vi "Финал (5).vi"(0 "Dec":T5, 1 "Cread":bool, 2 "adr A":cluster{"A1":bool, "A0":bool}, 3 "adr B":cluster{"B1":bool, "B0":bool}, 4 "SelInp":bool, 5 "C Func":T1, 6 "SelOp":bool, 7 "Reset Out":bool, 8 "WR":bool, 9 "Reset":bool, 10 "C":bool, 11 "Exec":bool, 12 "Reset Memory":bool, 13 "ClearAcc":bool, 19 "Read":bool) -> (14 "L":T3, 15 "Flags":T4, 16 "Digs":T2)   [LabVIEW 2017]
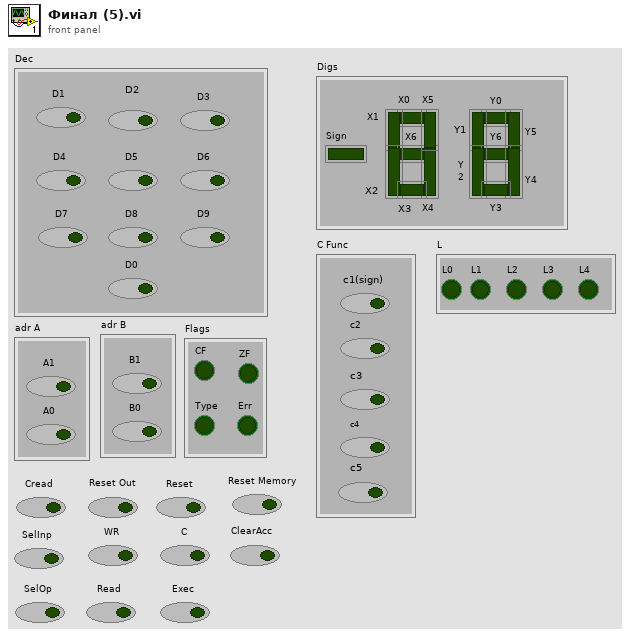
[diagram p1: front panel]
types:
  T1 = cluster{"c1(sign)":bool, "c2":bool, "c3":bool, "c4":bool, "c5":bool}
  T2 = cluster{"Y0":bool, "Y1":bool, "Y5":bool, "Y6":bool, "Y\n2":bool, "Y4":bool, "Y3":bool, "X0":bool, "X1":bool, "X6":bool, "X4":bool, "X2":bool, "X5":bool, "X3":bool, "Sign":bool}
  T3 = cluster{"L0":bool, "L1":bool, "L2":bool, "L3":bool, "L4":bool}
  T4 = cluster{"CF":bool, "ZF":bool, "Type":bool, "Err":bool}
  T5 = cluster{"D0":bool, "D1":bool, "D2":bool, "D3":bool, "D4":bool, "D5":bool, "D6":bool, "D7":bool, "D8":bool, "D9":bool}
  T6 = cluster{"b 0":bool, "b 1":bool, "b 2":bool, "b 3":bool, "b 4":bool}
  T7 = cluster{"q 1":bool, "q 2":bool, "q 3":bool, "q 4":bool, "q 5":bool}
  T8 = cluster{"q 0":bool, "q 1":bool, "q 2":bool, "q 3":bool, "q 4":bool}
  T9 = cluster{"B 0":bool, "B 1":bool, "B 2":bool, "B 3":bool, "B 4":bool}
  T10 = cluster{"A 0":bool, "A 1":bool, "A 2":bool, "A 3":bool, "A 4":bool}
  T11 = cluster{"CF":bool, "ZF":bool, "Type":bool, "ERROR":bool}
  T12 = cluster{"y0":bool, "y1":bool, "y5":bool, "y6":bool, "y2":bool, "y4":bool, "y3":bool, "x 0":bool, "x 1":bool, "x 6":bool, "x 4":bool, "x 2":bool, "x 5":bool, "x 3":bool, "Sign":bool}
  T13 = cluster{"x 0":bool, "x 1":bool, "x 2":bool, "x 3":bool, "x 4":bool}
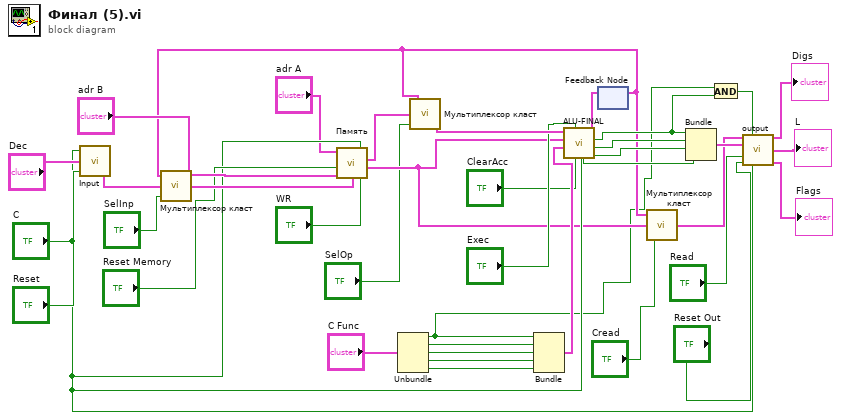
[diagram p0: block diagram]
diagram:
  n1 = call "Input.vi"("Reset"="Reset", "Dec"="Dec", "C"="C") -> ("Bin"=w5:T6)  [unwired: 1 in, 1 out]
  n2 = Unbundle("C Func") -> ("c1(sign)"=w3:bool, "c2"=w17:bool, "c3"=w16:bool, "c4"=w15:bool, "c5"=w14:bool)
  n3 = Bundle("c1(sign)"=w3, "c2"=w17, "c3"=w16, "c4"=w15, "c5"=w14) -> (w13:T1)  [unwired: 1 in]
  n4 = feedback #1() -> (w7:T7)  [unwired: 1 in]
  n5 = call "Мультиплексор класт.vi"("МХ"="SelInp", "Cl 0"=w5, "Cl 1"=w7) -> ("cl 2"=w35:T8)
  n6 = call "Память.vi"("WR"="WR", "C"="C", "adr B"="adr B", "RESET"="Reset Memory", "Cluster d"=w35, "Adr A"="adr A") -> ("out B"=w6:T9, "out A"=w31:T10)
  n7 = call "Мультиплексор класт.vi"("МХ"="SelOp", "Cl 0"=w31, "Cl 1"=w7) -> ("cl 2"=w30:T8)
  n8 = call "ALU-FINAL.vi"("Reset Button"="ClearAcc", 6:"Exec", 7:"C"="C", 8:"C"=w13, "B"=w6, "A"=w30) -> ("Type"=w28:bool, "ZF"=w29:bool, "CF"=w12:bool, "Q"=w25:T7, "ERROR"=w27:bool)
  n9 = feedback-in #1(w25) -> ()
  n10 = call "Мультиплексор класт.vi"("МХ"="Cread", "Cl 0"=w6, "Cl 1"=w7) -> ("cl 2"=w23:T8)
  n11 = Bundle("CF"=w12, "ZF"=w29, "Type"=w28, "ERROR"=w27) -> (w24:T11)  [unwired: 1 in]
  n12 = And(x=w3, y=w12) -> (x .and. y?=w11:bool)
  n13 = call "output.vi"("Bin_I"=w23, "sign"=w11, "flags_I"=w24, "C"="C", "Read"="Read", "Reset"="Reset Out") -> ("Digitals"=→"Digs":T12, "Bin_O"=→"L":T13, "Flags_O"=→"Flags":T4)  [unwired: 7 in]
